vi "parse_retrieve_arrayof_point_response.vi"(8 "error in (no error)":errorcluster, 10 "body":string, 11 "headers":string) -> (0 "error out":errorcluster, 3 "Array":T1[](array[typedef]))   [LabVIEW 2020, in "vector_qdrant.lvclass"]
uses:
  vector_qdrant.lvclass
  abstract_vector_base/vector.ctl
  abstract_vector_base/abstract_vector_base.lvclass
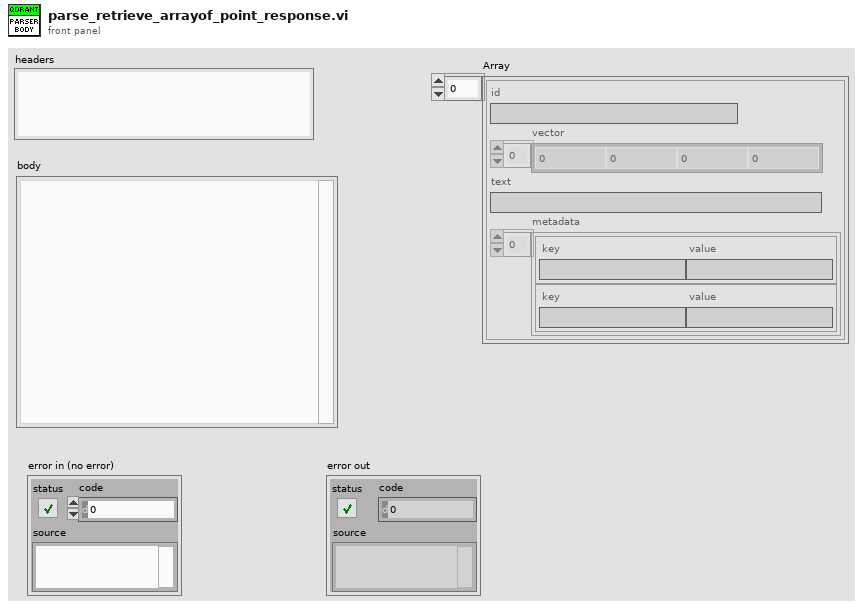
[diagram p1: front panel]
types:
  T1 = typedef "abstract_vector_base.lvclass/vector.ctl" = cluster{"id":string, "vector":dbl[], "text":string, "metadata":cluster{"key":string, "value":string}[]}
  T2 = cluster{"id":string, "payload":cluster{"text":string}, "vector":dbl[]}[]
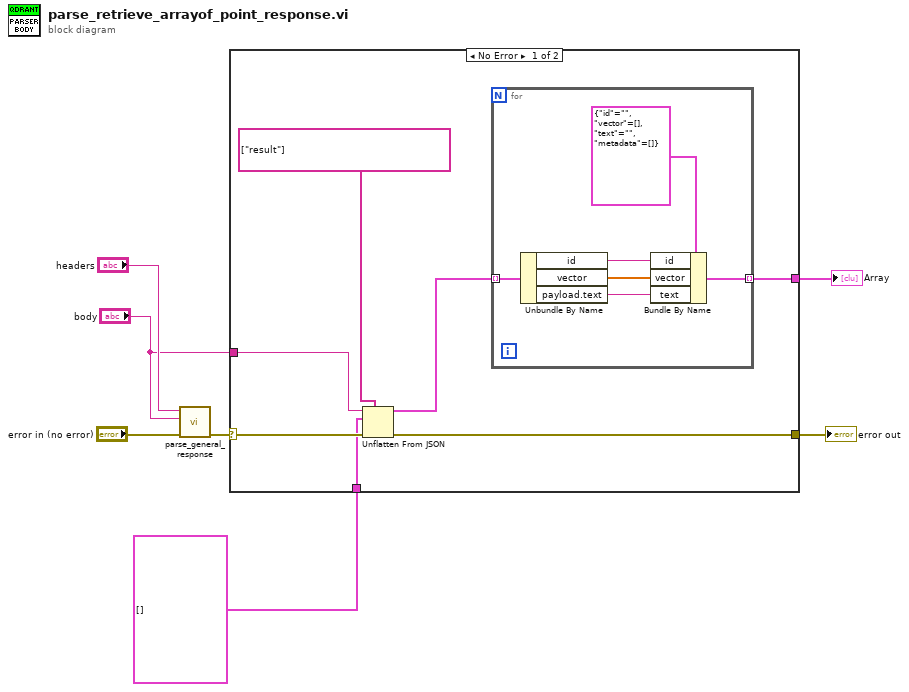
[diagram p0: block diagram]
diagram:
  n1 = call "parse_general_response.vi"("error in (no error)"="error in (no error)", "body"="body", "headers"="headers") -> ("error out"=w5:errorcluster)  [unwired: 8 in]
  n2 = case shown="No Error" w5 {
    selector: w5 -> [w14 w21]
    tunnel: [w11 w21] -> w7
    tunnel: "body" -> [w12 _]
    tunnel: T2 [] -> [w10 _]
    tunnel: [w8 _] -> w2
    frame No Error {
      n3 = Unflatten From JSON(path=string[] ["result"], JSON string=w12, type and defaults=w10, error in (no error)=w14) -> (value=w9:T2, error out=w11:errorcluster)  [unwired: 3 in]
      n4 = for {
        tunnel: w9 -> [w20] mode=indexing
        tunnel: [w19] -> w8 mode=indexing
        n5 = Unbundle By Name(w20) -> ("id"=w18:string, "vector"=w17:dbl[], "payload.text"=w16:string)
        n6 = Bundle By Name(cluster=T1 {"id"="", "vector"=[], "text"="", "metadata"=[]} ("vector"), "id"=w18, "vector"=w17, "text"=w16) -> (w19:T1)
      }
    }
    frame Error {
    }
  }
  "error out" <- w7
  "Array" <- w2
